vi "JoystickRecieve.vi"(8 "error in (no error)":errorcluster, 11 "Notifier Name":string="Joystick") -> (0 "error out":errorcluster, 3 "notification":T1)   [LabVIEW 2013]
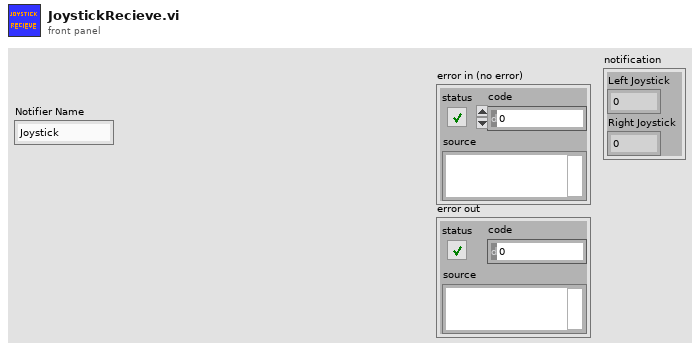
[diagram p1: front panel]
types:
  T1 = cluster{"Left Joystick":dbl, "Right Joystick":dbl}
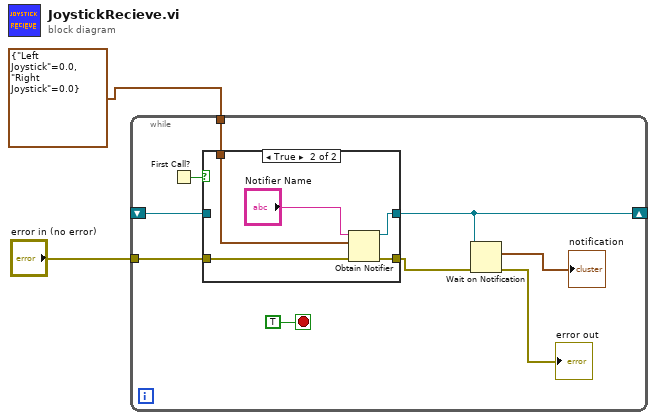
[diagram p0: block diagram]
diagram:
  n1 = while {
    shift-right: [w7] -> _
    shift-left: _ -> [w8]
    tunnel: "error in (no error)" -> [w9]
    tunnel: T1 {"Left Joystick"=0.0, "Right Joystick"=0.0} -> [w4]
    stop <- TRUE stop-if-true
    n2 = First Call?() -> (First Call?: T/F=w10:bool)
    n3 = case shown="True" w10 {
      tunnel: [w13 w16] -> w7
      tunnel: w9 -> [w12 w17]
      tunnel: w8 -> [w13 _]
      tunnel: [w12 w15] -> w6
      tunnel: w4 -> [_ w14]
      frame False {
      }
      frame True {
        n4 = Obtain Notifier(name (unnamed)="Notifier Name", notification data type=w14, error in (no error)=w17) -> (notifier out=w16:refnum<notifier>, error out=w15:errorcluster)  [unwired: 1 in, 1 out]
      }
    }
    n5 = Wait on Notification(notifier=w7, error in (no error)=w6) -> (notification=→"notification":T1, error out=→"error out":errorcluster)  [unwired: 2 in, 2 out]
  }
